vi "Agilent PWM Read Zeroing Type.vi"(7 "Agilent PWM":T1, 8 "error in (no error)":errorcluster, 11 "VISA Resource Name":refnum<visa-resource-name>) -> (0 "error out":errorcluster, 2 "Frequency (MHz)":enum16{"Internal", "External"}(ring), 3 "dup VISA Resource Name":refnum<visa-resource-name>)   [LabVIEW 2011]
doc: "This VI for the HP 8753 is used to read the sweep type.\n\n0 LINEAR FREQ\n1 LOG FREQ\n2 LIST FREQ\n3 CW TIME\n4 POWER SWEEP"
uses:
  TypeDefs/Agilent PWM Instrument Info.ctl
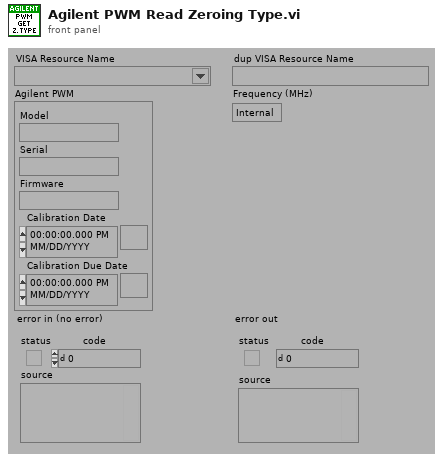
[diagram p1: front panel]
types:
  T1 = typedef "Agilent PWM Instrument Info.ctl" = cluster{"Model":string, "Serial":string, "Firmware":string, "Calibration Date":timestamp, "Calibration Due Date":timestamp}
  T2 = typedef "Agilent PWM Model.ctl" = enum16{"Not Supported", "E4418X", "E4419X", "U2000X"}
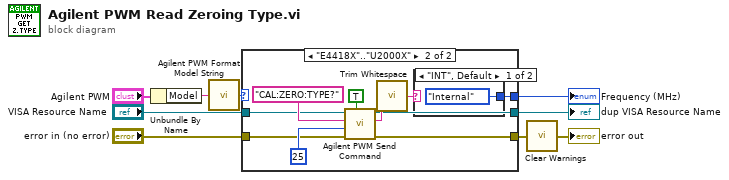
[diagram p0: block diagram]
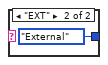
[diagram p3: hidden frame]
diagram:
  n1 = Unbundle By Name("Agilent PWM") -> ("Model"=w2:string)
  n2 = call "Agilent PWM Format Model String.vi"("Model"=w2) -> ("Model"=w1:T2)
  n3 = case shown="\"E4418X\"..\"U2000X\"" w1 {
    tunnel: [w11 w20] -> w9
    tunnel: "VISA Resource Name" -> [w10 w16]
    tunnel: "error in (no error)" -> [w11 w15]
    tunnel: [w10 w14] -> w5
    tunnel: [_ w12] -> w4
    frame "Not Supported", Default {
    }
    frame "E4418X".."U2000X" {
      n4 = call "Agilent PWM Send Command.vi"("Read? (F)"=TRUE, "error in (no error)"=w15, "Byte Count"=u32 25, "Command"="CAL:ZERO:TYPE?" ("write buffer"), "VISA Resource Name"=w16) -> ("error out"=w20:errorcluster, "Data Read"=w17:string, "dup VISA Resource Name"=w14:refnum<visa-resource-name>)  [unwired: 4 out]
      n5 = call <vilib>:"Trim Whitespace.vi"("string"=w17) -> ("trimmed string"=w13:string)  [unwired: 1 in]
      n6 = case shown="\"INT\", Default" w13 {
        tunnel: [enum16{"Internal", "External"}."Internal" ("Frequency (MHz)") enum16{"Internal", "External"}."External" ("Frequency (MHz)")] -> w12
        frame "INT", Default {
        }
        frame "EXT" {
        }
      }
    }
  }
  "dup VISA Resource Name" <- w5
  "Frequency (MHz)" <- w4
  n7 = call "Clear Warnings.vi"("error in (no error)"=w9) -> ("error out"=→"error out":errorcluster)
